vi "Find Fire Symbol.vi"(0 "Image In":T1, 5 "Image Dst":T1, 7 "Template File Path":path=path "C:/Users/EISD/Desktop/SVN Internal/Robot/Programming/Competition Code/cRIO Project/fire geo template super scale.png", 11 "error in":errorcluster) -> (3 "Matches (Geometric Matching 1)":T2[](array[typedef]) {"Correlation Score" format="%.2f"; "Target Template Curve Score" format="%.2f"; "Template Target Curve Score" format="%.2f"; "Bounding Box"."y" format="%.2f"; "Bounding Box"."x" format="%.2f"; "Position"."y" format="%.2f"; "Position"."x" format="%.2f"; "Score" format="%.2f"; "Scale" format="%.2f"; "Angle" format="%.2f"; "Occlusion %" format="%.2f"}, 4 "Image Out":T1, 6 "Number of Matches (Geometric Matching 1)":i32, 15 "error out":errorcluster)   [LabVIEW 2013]
uses:
  <vilib>/vision/Image Controls.llb/IMAQ Image.ctl
  <vilib>/vision/Pattern Matching.llb/IMAQ GM Match Report.ctl
  <vilib>/vision/Pattern Matching.llb/IMAQ Curve Parameters.ctl
  <vilib>/vision/Pattern Matching.llb/IMAQ Match Range Setting.ctl
  <vilib>/vision/NI_Vision_Development_Module.lvlib
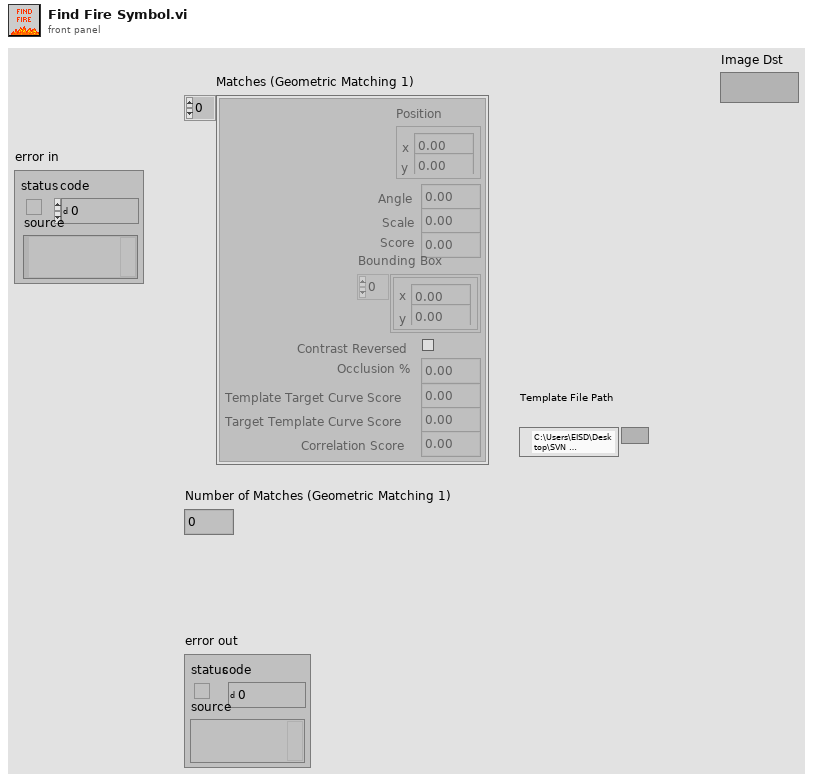
[diagram p1: front panel]
types:
  T1 = typedef "IMAQ Image.ctl" = refnum<image>
  T2 = typedef "IMAQ GM Match Report.ctl" = cluster{"Position":cluster{"x":sgl, "y":sgl}, "Angle":sgl, "Scale":sgl, "Score":sgl, "Bounding Box":cluster{"x":sgl, "y":sgl}[], "Contrast Reversed":bool, "Occlusion %":sgl, "Template Target Curve Score":sgl, "Target Template Curve Score":sgl, "Correlation Score":sgl}
  T3 = typedef "IMAQ Curve Parameters.ctl" = cluster{"Extraction Mode":u32, "Edge Threshold":i32, "Edge Filter Size":u32, "Min Length":i32, "Row Search Step Size":i32, "Col Search Step Size":i32, "Max Endpoint Gap":i32, "Closed":bool, "Subpixel":bool}
  T4 = typedef "IMAQ Match Range Setting.ctl" = cluster{"Match Constraints":u32, "Min":dbl, "Max":dbl}
  T5 = cluster{"Curve Parameters":T3, "Match Mode":cluster{"Rotation":bool, "Scale":bool, "Occlusion":bool, "Reserved":bool, "Reserved":bool, "Reserved":bool}, "Range Settings":T4[], "Number of Matches":i32, "Minimum Match Score":sgl, "SubPixel Accuracy":bool, "Adv. Geometric Match Options 2":cluster{"Setup Data Item":u16, "Item Value":dbl}[]}
  T6 = cluster{"Global Rectangle":i32[], "Contours":cluster{"ID":enum32{"External", "Internal"}, "Type":u32, "Coordinates":i32[]}[]}
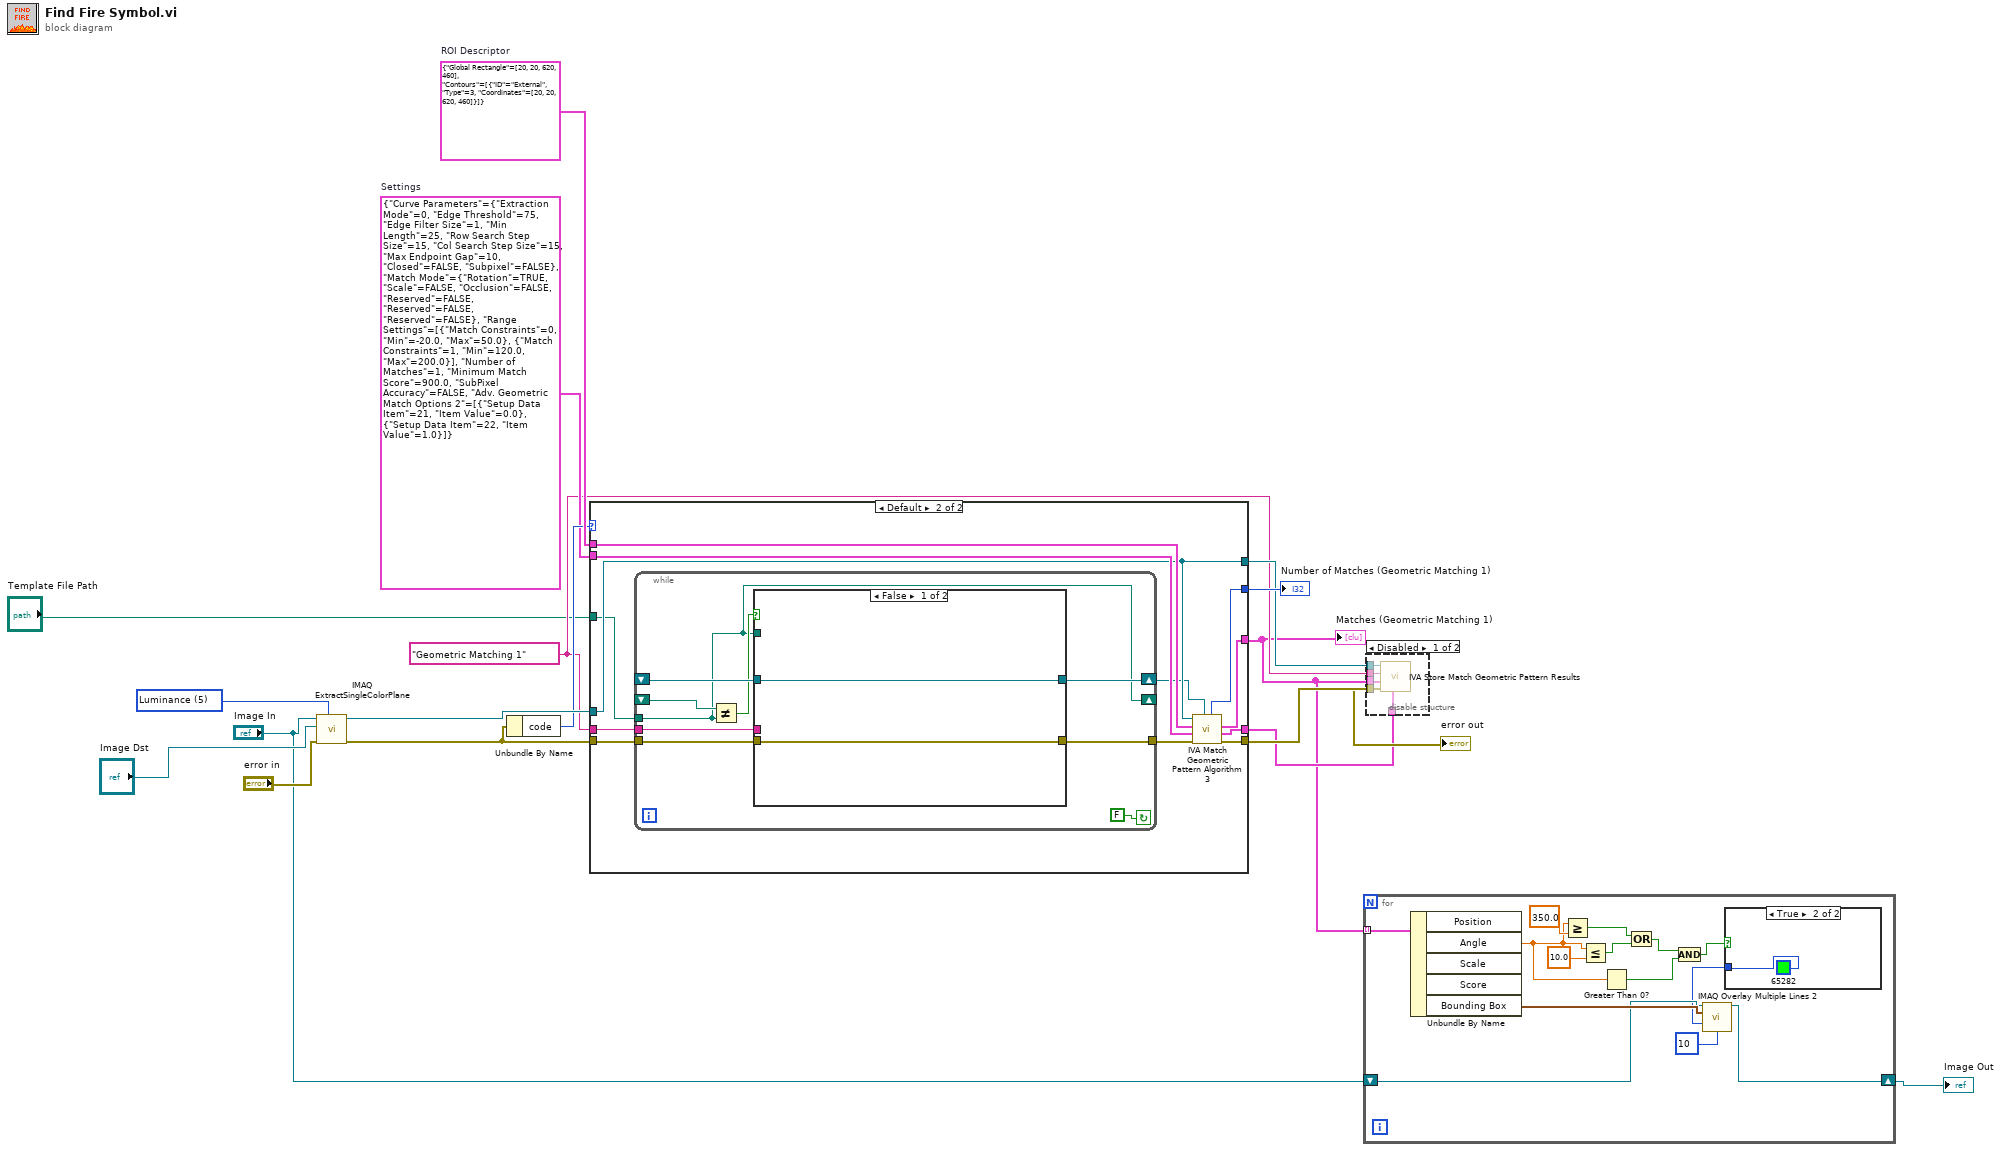
[diagram p0: block diagram]
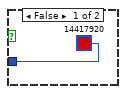
[diagram p3: hidden frame]
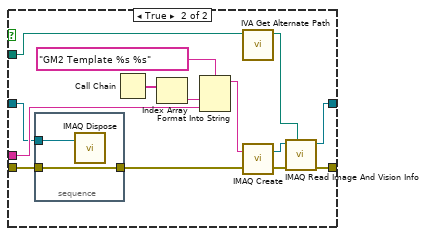
[diagram p5: hidden frame]
diagram:
  w7 = T5 {"Curve Parameters"={"Extraction Mode"=0, "Edge Threshold"=75, "Edge Filter Size"=1, "Min Length"=25, "Row Search Step Size"=15, "Col Search Step Size"=15, "Max Endpoint Gap"=10, "Closed"=FALSE, "Subpixel"=FALSE}, "Match Mode"={"Rotation"=TRUE, "Scale"=FALSE, "Occlusion"=FALSE, "Reserved"=FALSE, "Reserved"=FALSE, "Reserved"=FALSE}, "Range Settings"=[{"Match Constraints"=0, "Min"=-20.0, "Max"=50.0}, {"Match Constraints"=1, "Min"=120.0, "Max"=200.0}], "Number of Matches"=1, "Minimum Match Score"=900.0, "SubPixel Accuracy"=FALSE, "Adv. Geometric Match Options 2"=[{"Setup Data Item"=21, "Item Value"=0.0}, {"Setup Data Item"=22, "Item Value"=1.0}]}  # Settings
  w6 = "Geometric Matching 1" ("Step Name")
  w16 = T6 {"Global Rectangle"=[20, 20, 620, 460], "Contours"=[{"ID"=enum."External", "Type"=3, "Coordinates"=[20, 20, 620, 460]}]}  # ROI Descriptor
  w18 = 5 items=["Red", "Green", "Blue", "Hue", "Saturation", "Luminance", "Value", "Intensity"] ("Color Plane")
  n1 = call "IMAQ ExtractSingleColorPlane"("Color Plane"=w18, "error in (no error)"="error in", "Image Dst"="Image Dst", "Image Src"="Image In") -> ("error out"=w10:errorcluster, "Image Dst Out"=w15:T1)  [unwired: 6 out]
  n2 = Unbundle By Name(w10) -> ("code"=w9:i32)
  n3 = case shown="Default" w9 {
    tunnel: "Template File Path" -> [_ w21]
    tunnel: w10 -> [_ w22]
    tunnel: w7 -> [_ w31]
    tunnel: w16 -> [_ w30]
    tunnel: w15 -> [w19 w25]
    tunnel: [_ w29] -> w14
    tunnel: [_ w28] -> w4
    tunnel: [_ w27] -> w12
    tunnel: [_ w26] -> w11
    tunnel: [w19 w25] -> w8
    tunnel: w6 -> [_ w20]
    frame -1074396199, -1074396198 {
      # "Discard Coordinate System Error"
    }
    frame Default {
      n4 = while {
        shift-right: [w40] -> w23
        shift-left: _ -> [w39]
        tunnel: [w37] -> w24
        tunnel: w22 -> [w36]
        tunnel: w21 -> [w32]
        tunnel: w20 -> [w35]
        shift-right: [w32] -> _
        shift-left: _ -> [w34]
        stop <- FALSE continue-if-true
        n5 = Not Equal?(x=w34, y=w32) -> (x != y?=w33:bool)
        n6 = case shown="False" w33 {
          tunnel: [w42 w54] -> w40
          tunnel: w39 -> [w42 w46]
          tunnel: [w41 w51] -> w37
          tunnel: w36 -> [w41 w47]
          tunnel: w35 -> [_ w48]
          tunnel: w32 -> [_ w44]
          frame False {
          }
          frame True {
            n7 = stacked-sequence {
              tunnel: w47 -> [w58]
              tunnel: w46 -> [w57]
              tunnel: [w58] -> w45
              frame #0 {
                n8 = call "IMAQ Dispose"("Image"=w57) -> ()  [unwired: 2 in, 4 out]
              }
            }
            n9 = Call Chain() -> (call chain=w50:string[])
            n10 = Index Array(array=w50) -> (element=w49:string)  [unwired: 1 in]
            n11 = Format Into String(format string="GM2 Template %s %s" ("Image Name"), w49, w48) -> (resulting string=w56:string)  [unwired: 2 in, 1 out]
            n12 = call <vilib>:"IVA Get Alternate Path.vi"("Path In"=w44) -> ("Path Out"=w43:path)  [unwired: 10 out]
            n13 = call "IMAQ Create"("Image Name"=w56, "error in (no error)"=w45) -> ("New Image"=w53:T1, "error out"=w52:errorcluster)  [unwired: 2 in, 1 out]
            n14 = call "IMAQ Read Image And Vision Info"("File Path"=w43, "error in (no error)"=w52, "Image"=w53) -> ("error out"=w51:errorcluster, "Image Out"=w54:T1)  [unwired: 1 in, 6 out]
          }
        }
      }
      n15 = call <vilib>:"IVA Match Geometric Pattern Algorithm 3.vi"("Template"=w23, "error in (no error)"=w24, "Settings"=w31, "ROI Descriptor"=w30, "Image"=w25) -> ("error out"=w29:errorcluster, "Calibrated Matches"=w27:T2[], "Matches"=w28:T2[], "Number of Matches"=w26:i32)  [unwired: 3 out]
    }
  }
  "Matches (Geometric Matching 1)" <- w4
  "Number of Matches (Geometric Matching 1)" <- w11
  n16 = for {
    tunnel: w4 -> [w72] mode=indexing
    shift-right: [w59] -> w2
    shift-left: "Image In" -> [w70]
    n17 = Unbundle By Name(w72) -> ("Angle"=w67:sgl, "Bounding Box"=w71:cluster{"x":sgl, "y":sgl}[])  [unwired: 3 out]
    n18 = Greater Or Equal?(x=w67, y=sgl 350.0) -> (x >= y?=w65:bool)
    n19 = Less Or Equal?(x=w67, y=sgl 10.0) -> (x <= y?=w64:bool)
    n20 = Greater Than 0?(x=w67) -> (x > 0?=w62:bool)
    n21 = Or(x=w65, y=w64) -> (x .or. y?=w63:bool)
    n22 = And(x=w63, y=w62) -> (x .and. y?=w61:bool)
    n23 = case shown="True" w61 {
      tunnel: [u32 14417920 ("Color") u32 65282 ("Color")] -> w60
      frame False {
      }
      frame True {
      }
    }
    n24 = call "IMAQ Overlay Multiple Lines 2"("Image"=w70, "Line End Points"=w71, "Color"=w60, "Width"=u32 10) -> ("Image Out"=w59:T1)  [unwired: 10 in, 1 out]
  }
  "Image Out" <- w2
  n25 = disable-structure shown="Disabled" {
    disable-tunnel: w14 -> [w80 _]
    disable-tunnel: [w79 _] -> w13
    disable-tunnel: w12 -> [w78 _]
    disable-tunnel: w8 -> [w77 _]
    disable-tunnel: w6 -> [w76 _]
    disable-tunnel: w4 -> [w75 _]
    frame Disabled {
      n26 = call <vilib>:"IVA Store Match Geometric Pattern Results.vi"("Calibrated Matches"=w78, "error in (no error)"=w80, "Matches"=w75, "Step Name"=w76, "Image in"=w77) -> ("error out"=w79:errorcluster)  [unwired: 6 out]
    }
    frame Enabled {
    }
  }
  "error out" <- w13
